vi "Injection.DelayAndDigitalFilter.vi"(4 "Pretrigger Samples":u8=5, 6 "Cycles to Filter":u8=5, 8 "Active Edge":bool, 9 "Threshold":fxp<+/-,32,8>, 10 "Current (PreScaled)":fxp<+/-,32,8>, 11 "Voltage (PreScaled)":fxp<+/-,32,8>) -> (1 "Output Filtered Signal":bool, 2 "Current (PreScaled)":fxp<+/-,32,8>, 3 "Voltage (PreScaled)":fxp<+/-,32,8>)   [LabVIEW 2015]
uses:
  <vilib>/rvi/DataTransferAndStorage/Container/Common/niFpgaContainerGetUniqueNameForEmu.vi
  <vilib>/rvi/DataTransferAndStorage/Container/Common/niFpgaContainerSetEmuInfo.vi
  <vilib>/rvi/eio/common/nirviEmuReportErrorAndStop.vi
  <vilib>/rvi/DataTransferAndStorage/Container/Common/niFpgaContainerExecOnDevCompGetState.vi
  <vilib>/rvi/Emulation/niFpgaEmulationIsFPGAContextNoSignature.vi
  <vilib>/rvi/Emulation/niFpgaProcessEmulError.vi
  <vilib>/rvi/Emulation/niFpgaSctlEmulationGetInTimedLoop.vi
  <vilib>/rvi/errors/nirviReportUnexpectedCaseInternalError (U32).vi
  <vilib>/rvi/Memory/Memory_Emulation/niFpgaMemoryEmulationCacheClearOnFirstRun.vi
  <vilib>/rvi/Memory/Memory_Emulation/nirvimemoryEmulationManagerCache_MakeExclusive.vi
  <vilib>/rvi/Memory/Memory_Emulation/niFpgaMemoryEmulationValidateCache.vi
  <vilib>/rvi/Memory/Memory_Emulation/nirvimemoryEmulationManagerCache_InsertValue.vi
  <vilib>/Utility/error.llb/Clear Errors.vi
  <vilib>/rvi/Memory/Memory_Emulation/nirvimemoryEmulationManagerCache_ReleaseExclusive.vi
  <vilib>/rvi/Memory/Memory_Emulation/nirvimemoryEmulationManagerCache_GetValue.vi
  <vilib>/rvi/Memory/Memory_Emulation/nirvimemoryEmulationManagerCache_SetValue.vi
  <vilib>/rvi/Emulation/niFpgaSctlEmulationResourceMgr.vi
  <vilib>/rvi/LocalResourceManager/LocalResourceManager.xnode
  <vilib>/rvi/DataTransferAndStorage/Container/XNode/niFpgaContainer.xnode
  <vilib>/rvi/Memory/Memory_Emulation/niFpgaMemoryEmulationRefIn.vi
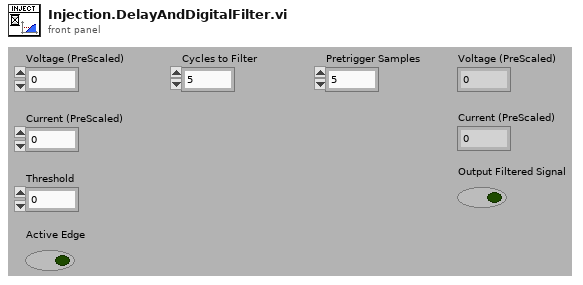
[diagram p1: front panel]
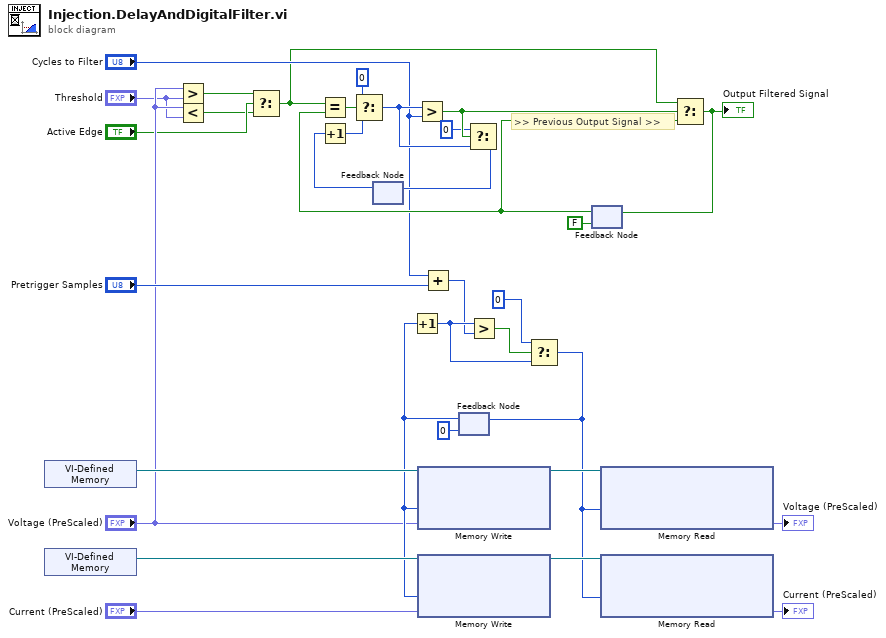
[diagram p0: block diagram]
diagram:
  # ">> Previous Output Signal >>"
  n1 = xnode "VI-Defined Memory"() -> ("Memory Out"=w20:refnum<k21>)
  n2 = xnode "VI-Defined Memory"() -> ("Memory Out"=w15:refnum<k21>)
  n3 = Greater?(x="Voltage (PreScaled)", y="Threshold") -> (0:w3:bool)
  n4 = Less?(x="Voltage (PreScaled)", y="Threshold") -> (x < y?=w1:bool)
  n5 = Select(t=w3, s="Active Edge", f=w1) -> (s? t:f=w2:bool)
  n6 = feedback #1() -> (w32:u8)  [unwired: 1 out]
  n7 = Increment(x=w32) -> (x+1=w28:u8)
  n8 = Add(x="Cycles to Filter", y="Pretrigger Samples") -> (x+y=w10:u8)
  n9 = feedback #2(u16 0 ("t")) -> (w14:u16)
  n10 = Increment(x=w14) -> (x+1=w22:u16)
  n11 = xnode "Memory Write"("Address"=w14, "Data"="Voltage (PreScaled)", "Memory In"=w20) -> ("Memory Out"=w19:refnum<k21>)
  n12 = xnode "Memory Write"("Address"=w14, "Data"="Current (PreScaled)", "Memory In"=w15) -> ("Memory Out"=w17:refnum<k21>)
  n13 = Greater?(x=w22, y=w10) -> (0:w23:bool)
  n14 = Select(t=u16 0, s=w23, f=w22) -> (s? t:f=w16:u16)
  n15 = feedback-in #2(w16) -> ()
  n16 = feedback #3(FALSE) -> (w30:bool)
  n17 = Equal?(x=w2, y=w30) -> (x = y?=w31:bool)
  n18 = Select(t=u8 0 ("f"), s=w31, f=w28) -> (s? t:f=w25:u8)
  n19 = Greater?(x=w25, y="Cycles to Filter") -> (0:w27:bool)
  n20 = Select(t=u8 0, s=w27, f=w25) -> (s? t:f=w26:u8)
  n21 = feedback-in #1(w26) -> ()
  n22 = xnode "Memory Read"("Address"=w16, "Memory In"=w19) -> ("Data"=→"Voltage (PreScaled)":fxp<+/-,32,8>)  [unwired: 1 out]
  n23 = xnode "Memory Read"("Address"=w16, "Memory In"=w17) -> ("Data"=→"Current (PreScaled)":fxp<+/-,32,8>)  [unwired: 1 out]
  n24 = Select(t=w2, s=w27, f=w30) -> (s? t:f=w33:bool)
  "Output Filtered Signal" <- w33
  n25 = feedback-in #3(w33) -> ()
